vi "Validate Header.vi"(9 "Single":bool, 11 "source":string) -> (1 "valid":bool, 2 "offset past":i32)   [LabVIEW 2020, in "Multi Error Cluster.lvlib"]
doc: "Determine if the error cluster is an encoded single, multi, or a legacy cluster."
uses:
  <vilib>/MultiError/TokenizeJSON/Multi Error Cluster.lvlib
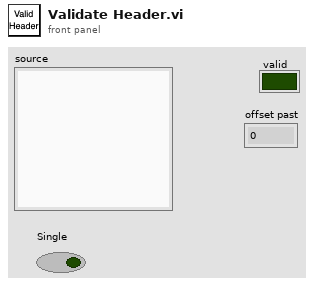
[diagram p1: front panel]
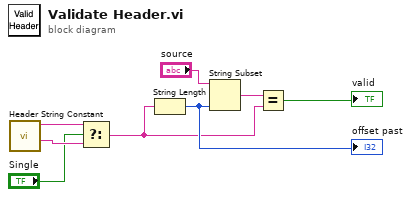
[diagram p0: block diagram]
diagram:
  n1 = call <vilib>:"Header String Constant.vi"() -> ("Multiple Header String"=w3:string, "Single Header String"=w4:string)  [unwired: 10 in]
  n2 = Select(t=w4, s="Single", f=w3) -> (s? t:f=w1:string)
  n3 = String Length(string=w1) -> (length=w8:i32)
  "offset past" <- w8
  n4 = String Subset(string="source", length (rest)=w8) -> (substring=w5:string)  [unwired: 1 in]
  n5 = Equal?(x=w5, y=w1) -> (x = y?=→"valid":bool)
